vi "Cache.Set Transfers Groups.vi"(10 "Transfers Groups":refnum<class "Transfer Group.lvclass">[](array[class]), 11 "Cache in":refnum<class "Cache.lvclass">) -> (3 "Cache out":refnum<class "Cache.lvclass">)   [LabVIEW 2017, in "DSF Core.lvlib" / "Cache.lvclass"]
uses:
  Cache.lvclass
  Transfer/Transfer Group.lvclass
  Cache.lvclass/Cache.ctl
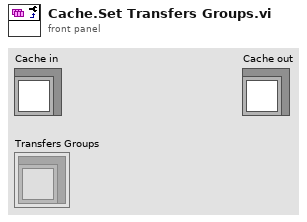
[diagram p1: front panel]
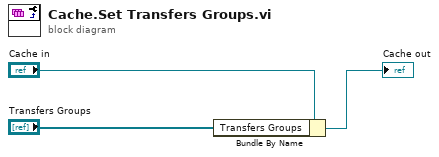
[diagram p0: block diagram]
diagram:
  n1 = Bundle By Name(cluster="Cache in", "Transfers Groups"="Transfers Groups") -> (→"Cache out":refnum<class "Cache.lvclass">)
